vi "Center Radius.vi"(10 "draw area cache in":T1) -> (1 "center":cluster{"horizontal":i16, "vertical":i16}, 2 "draw area cache out":T1, 4 "medium pen":T3, 5 "max radius":dbl, 6 "thick pen":T3)   [LabVIEW 2017, in "NI_Robotics_Compass Picture.lvlib"]
uses:
  <vilib>/robotics/Controls/Compass Indicator/Compass Picture/NI_Robotics_Compass Picture.lvlib
  <vilib>/robotics/Controls/Compass Indicator/Compass Picture/Draw Area State.ctl
  <vilib>/Utility/miscctls.llb/LVBoundsTypeDef.ctl
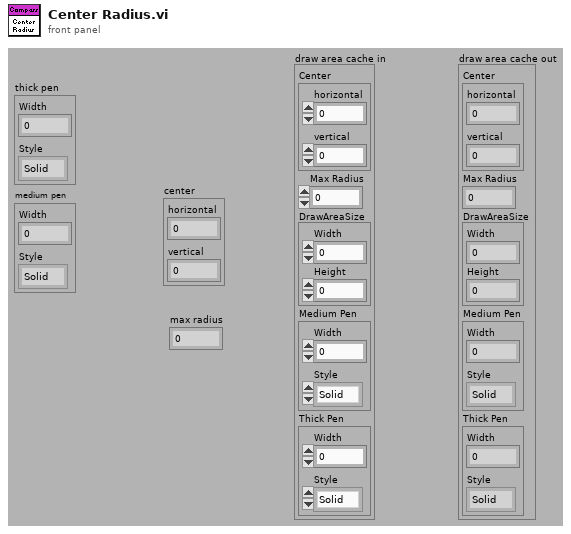
[diagram p1: front panel]
types:
  T1 = typedef "NI_Robotics_Compass Picture.lvlib/Draw Area State.ctl" = cluster{"Center":cluster{"horizontal":i16, "vertical":i16}, "Max Radius":dbl, "DrawAreaSize":T2, "Medium Pen":cluster{"Width":u16, "Style":enum32{"Solid", "Dash", "Dot", "DashDot", "DashDotDot"}}, "Thick Pen":cluster{"Width":u16, "Style":enum32{"Solid", "Dash", "Dot", "DashDot", "DashDotDot"}}}
  T2 = typedef "LVBoundsTypeDef.ctl" = cluster{"Width":u32, "Height":u32}
  T3 = cluster{"Width":u16, "Style":enum32{"Solid", "Dash", "Dot", "DashDot", "DashDotDot"}}
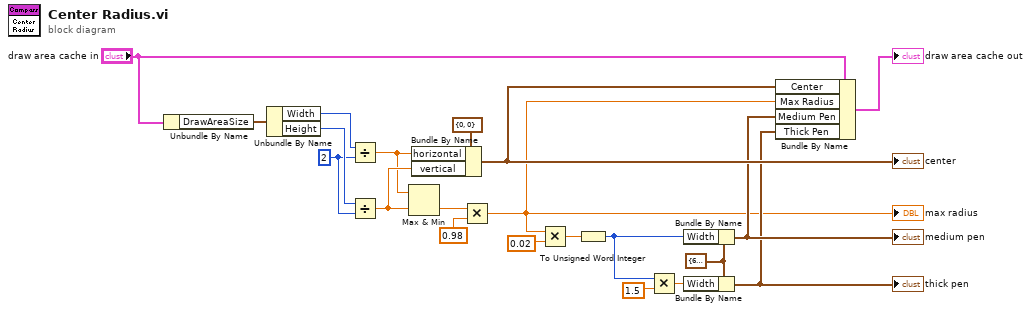
[diagram p0: block diagram]
diagram:
  w11 = u32 2 ("y")
  w21 = T3 {"Width"=6, "Style"=enum."Solid"} ("pen")
  n1 = Unbundle By Name("draw area cache in") -> ("DrawAreaSize"=w9:T2)
  n2 = Unbundle By Name(w9) -> ("Width"=w12:u32, "Height"=w13:u32)
  n3 = Divide(x=w12, y=w11) -> (x/y=w14:dbl)
  n4 = Divide(x=w13, y=w11) -> (x/y=w15:dbl)
  n5 = Max & Min(x=w14, y=w15) -> (min(x,y)=w3:dbl)  [unwired: 1 out]
  n6 = Bundle By Name(cluster=cluster{"horizontal":i16, "vertical":i16} {"horizontal"=0, "vertical"=0} ("pixel center"), "horizontal"=w14, "vertical"=w15) -> (w7:cluster{"horizontal":i16, "vertical":i16})
  "center" <- w7
  n7 = Multiply(x=w3, y=0.98) -> (x*y=w2:dbl)
  "max radius" <- w2
  n8 = Multiply(x=w2, y=0.02) -> (x*y=w19:dbl)
  n9 = To Unsigned Word Integer(number=w19) -> (unsigned 16bit integer=w17:u16)
  n10 = Multiply(x=w17, y=1.5) -> (x*y=w18:dbl)
  n11 = Bundle By Name(cluster=w21, "Width"=w17) -> (w5:T3)
  "medium pen" <- w5
  n12 = Bundle By Name(cluster=w21, "Width"=w18) -> (w4:T3)
  "thick pen" <- w4
  n13 = Bundle By Name(cluster="draw area cache in", "Center"=w7, "Max Radius"=w2, "Medium Pen"=w5, "Thick Pen"=w4) -> (→"draw area cache out":T1)
